vi "SubVI.vi"(8 "error in":errorcluster, 9 "Input3":bool, 10 "Input2":dbl, 11 "Input1":dbl) -> (0 "error out":errorcluster, 2 "Output2":string, 3 "Output1":string)   [LabVIEW 2020]
doc: "Use this template to build a VI to use as a subVI."
panel:
  # "Inputs"
  # "Outputs"
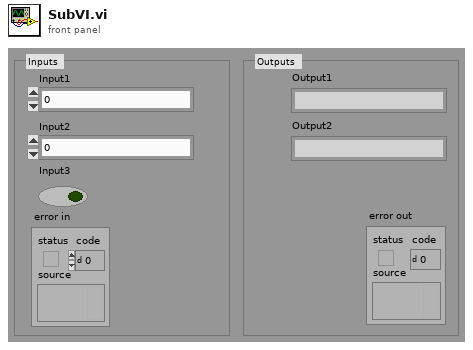
[diagram p1: front panel]
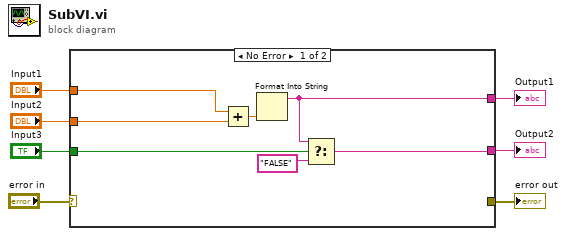
[diagram p0: block diagram]
diagram:
  n1 = case shown="No Error" "error in" {
    selector: "error in" -> [_ w15]
    tunnel: [_ w15] -> w6
    tunnel: "Input1" -> [w14 _]
    tunnel: "Input2" -> [w13 _]
    tunnel: [w11 _] -> w3
    tunnel: "Input3" -> [w10 _]
    tunnel: [w8 _] -> w1
    frame No Error {
      n2 = Add(x=w14, y=w13) -> (x+y=w12:dbl)
      n3 = Format Into String(w12) -> (resulting string=w11:string)  [unwired: 3 in, 1 out]
      n4 = Select(t=w11, s=w10, f="FALSE") -> (s? t:f=w8:string)
    }
    frame Error {
    }
  }
  "error out" <- w6
  "Output1" <- w3
  "Output2" <- w1
